vi "Read_Write_Local_table_Quick.vi"(3 "Mode":T1, 4 "String Values In":string[](array[string]), 5 "Ch names In":string[](array[string])) -> (0 "Numeric Values Out":dbl[](array[numeric]), 1 "String Values Out":string[](array[string]), 2 "Ch Names Out":string[](array[string]))   [LabVIEW 2020]
uses:
  ADAM Controls/Channel_names.ctl
  ADAM Controls/Quick_local_ADAM_Table.ctl
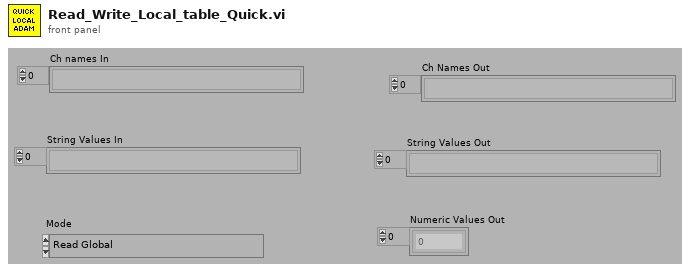
[diagram p1: front panel]
types:
  T1 = typedef "Quick_local_ADAM_Table.ctl" = enum16{"Read Global", "Load Global From ADAM Table", "Write Global"}
  T2 = typedef "Channel_names.ctl" = enum16{"Active Only", "Active + Off", "All Channels"}
  T3 = typedef "Ch_description_ADAM.ctl" = cluster{"Ch Name":string, "Type":T4, "Function":T5, "Ch State":T6, "Calibration type":T7, "A":dbl, "B":dbl, "C":dbl, "D":dbl, "Comments":string, "Address":T8, "String":string, "Duty":u16}
  T4 = typedef "Module_type_ADAM.ctl" = string
  T5 = typedef "Function_ADAM.ctl" = enum16{"Analogue Input", "Digital Input", "Event counter", "Event rate", "Analogue Output", "Digital Output", "Relay Output"}
  T6 = typedef "Channel_State.ctl" = enum16{"On", "Off", "Always On", "Always Off"}
  T7 = typedef "Calib_type_ADAM.ctl" = string
  T8 = typedef "Address.ctl" = cluster{"Main":i32, "Ch.":i32, "Sub":i32, "Port Name":string}
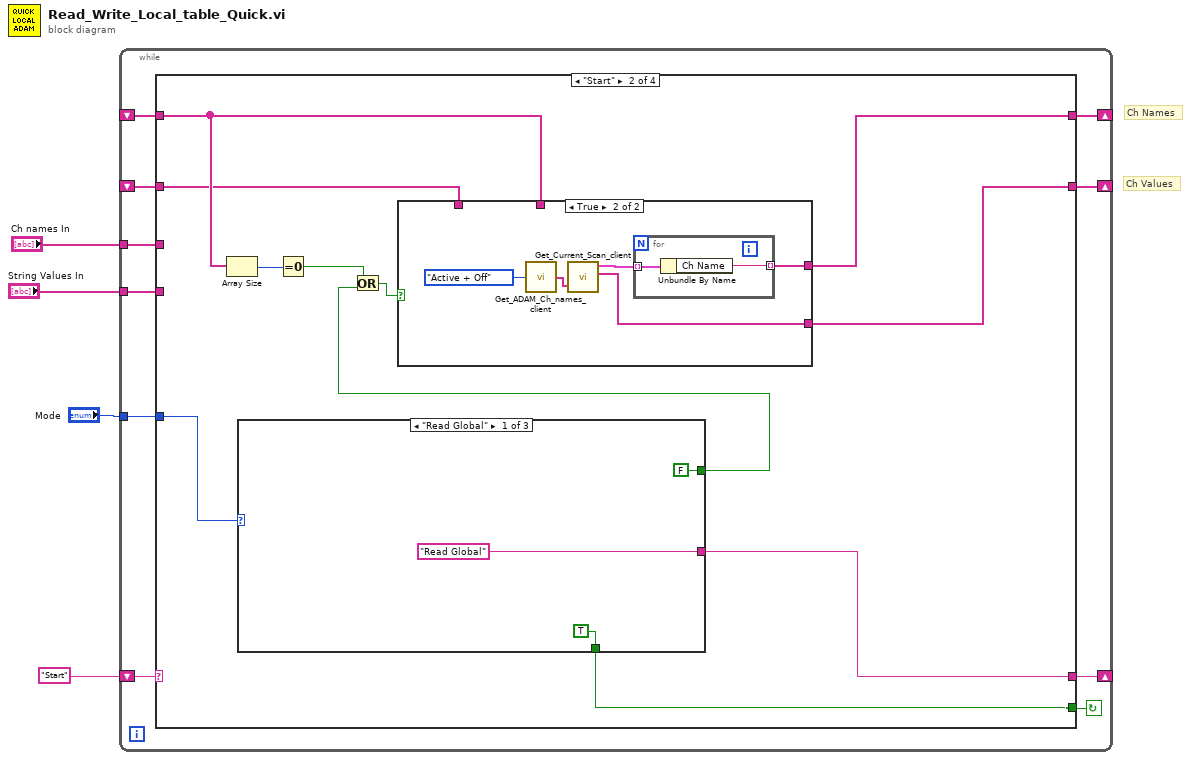
[diagram p0: block diagram]
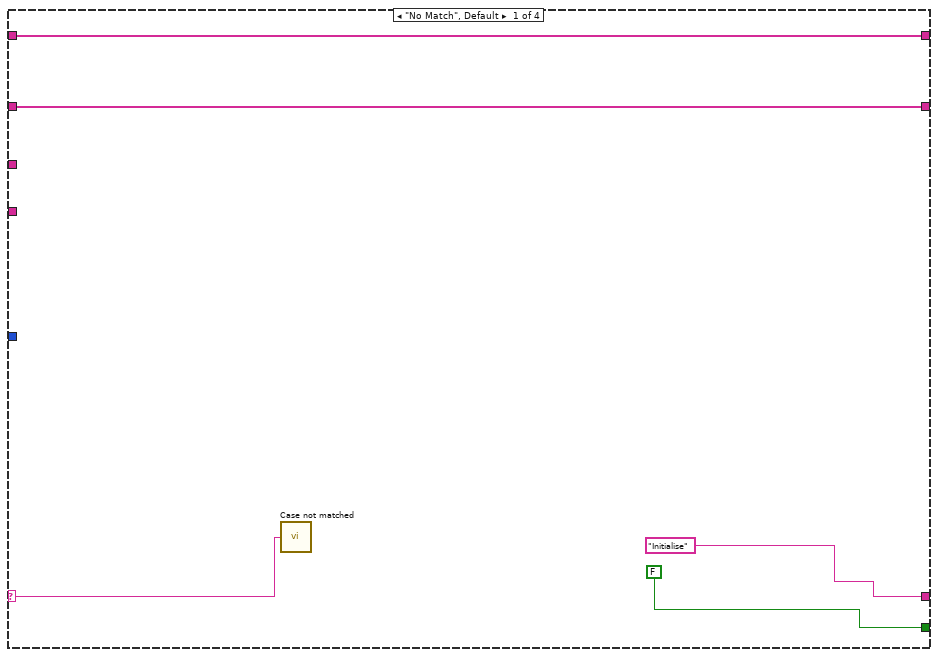
[diagram p2: hidden frame]
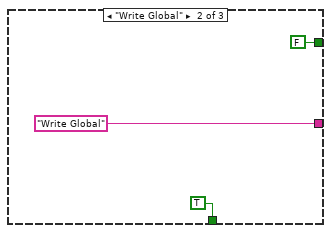
[diagram p4: hidden frame]
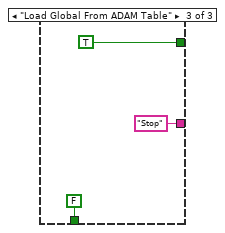
[diagram p5: hidden frame]
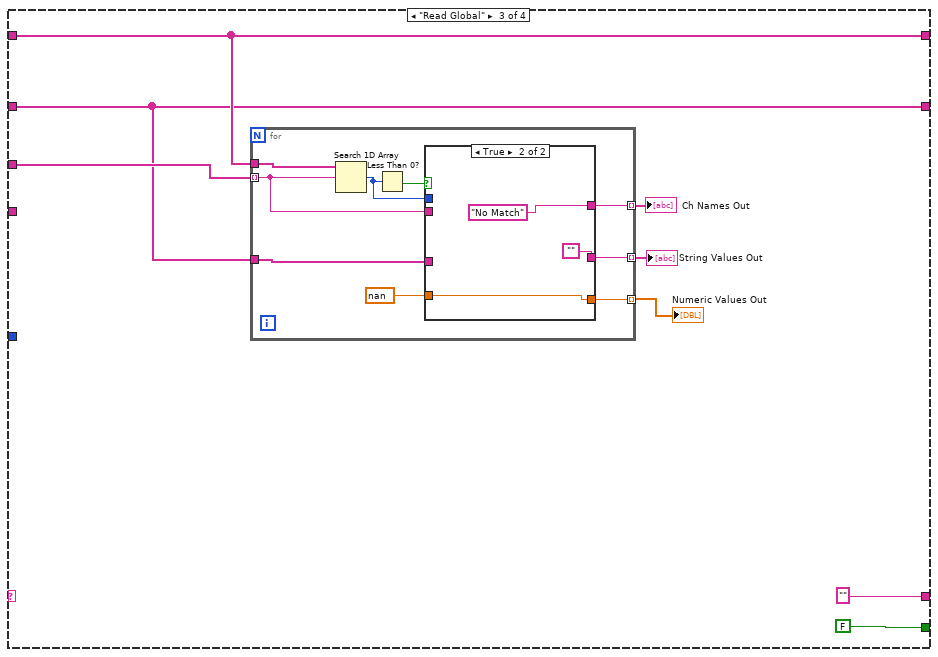
[diagram p6: hidden frame]
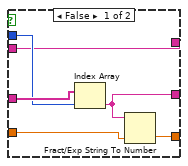
[diagram p7: hidden frame]
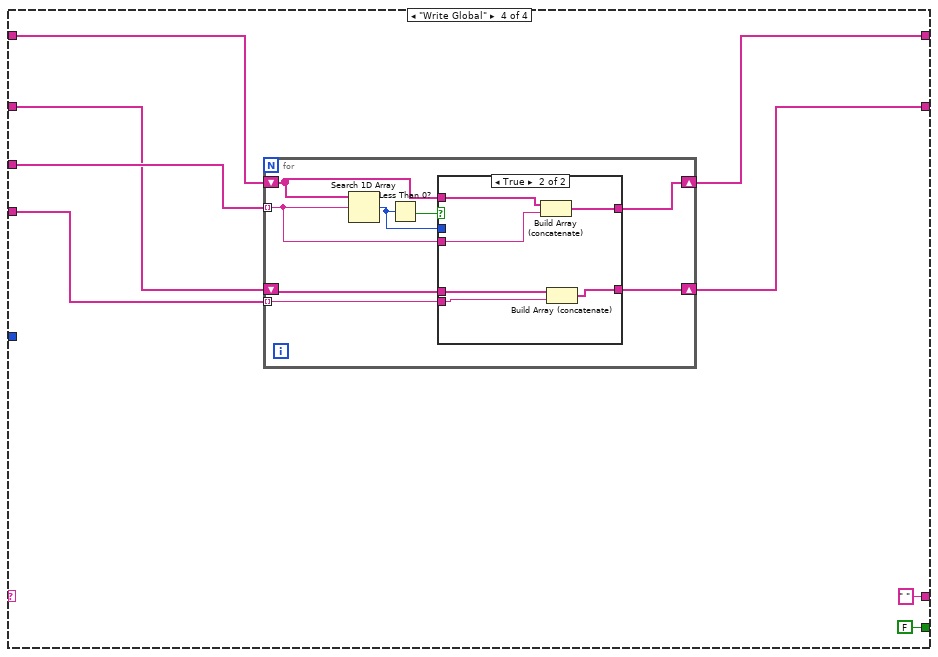
[diagram p8: hidden frame]
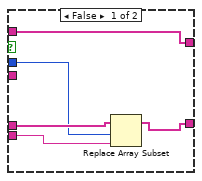
[diagram p9: hidden frame]
diagram:
  # "Ch Values"
  # "Ch Names"
  n1 = while {
    shift-left: "Start" -> [w12]
    shift-right: [w13] -> _
    shift-right: [w10] -> _
    shift-left: _ -> [w11]
    shift-right: [w9] -> _
    shift-left: _ -> [w7]
    tunnel: "Mode" -> [w8]
    tunnel: "Ch names In" -> [w6]
    tunnel: "String Values In" -> [w5]
    stop <- w14 continue-if-true
    n2 = case shown="\"Start\"" w12 {
      selector: w12 -> [w15 _ _ _]
      tunnel: [FALSE w20 FALSE FALSE] -> w14
      tunnel: ["Initialise" w21 "" " "] -> w13
      tunnel: w11 -> [w17 w23 w51 w82]
      tunnel: [w17 w30 w51 w80] -> w10
      tunnel: [w16 w29 w49 w77] -> w9
      tunnel: w8 -> [_ w28 _ _]
      tunnel: w7 -> [w16 w22 w49 w78]
      tunnel: w6 -> [_ _ w50 w81]
      tunnel: w5 -> [_ _ _ w79]
      frame "No Match", Default {
        n3 = call "Case not matched.vi"("Case Name not Matched"=w15) -> ()
      }
      frame "Start" {
        n4 = Array Size(array=w23) -> (size(s)=w27:i32)
        n5 = case shown="\"Read Global\"" w28 {
          tunnel: [FALSE FALSE TRUE] -> w26
          tunnel: ["Read Global" "Write Global" "Stop"] -> w21
          tunnel: [TRUE TRUE FALSE] -> w20
          frame "Read Global" {
          }
          frame "Write Global" {
          }
          frame "Load Global From ADAM Table" {
          }
        }
        n6 = Equal To 0?(x=w27) -> (x = 0?=w25:bool)
        n7 = Or(x=w25, y=w26) -> (x .or. y?=w24:bool)
        n8 = case shown="True" w24 {
          tunnel: [w32 w34] -> w30
          tunnel: [w31 w33] -> w29
          tunnel: w23 -> [w32 _]
          tunnel: w22 -> [w31 _]
          frame False {
          }
          frame True {
            n9 = call "Get_ADAM_Ch_names_client.vi"("Channel names set"=Channel_names."Active + Off") -> ("Ch names"=w36:string[])
            n10 = call "Get_Current_Scan_client.vi"("multipleChannels"=w36) -> ("Ch Description Array"=w37:T3[], "String values"=w33:string[])  [unwired: 2 in, 1 out]
            n11 = for {
              tunnel: w37 -> [w39] mode=indexing
              tunnel: [w38] -> w34 mode=indexing
              n12 = Unbundle By Name(w39) -> ("Ch Name"=w38:string)
            }
          }
        }
      }
      frame "Read Global" {
        n13 = for {
          tunnel: w50 -> [w64] mode=indexing
          tunnel: w49 -> [w62]
          tunnel: w51 -> [w61]
          tunnel: [w60] -> w52 mode=indexing
          tunnel: [w59] -> w53 mode=indexing
          tunnel: [w58] -> w54 mode=indexing
          n14 = Search 1D Array(1D array=w61, element=w64) -> (index of element=w63:i32)  [unwired: 1 in]
          n15 = Less Than 0?(x=w63) -> (x < 0?=w65:bool)
          n16 = case shown="True" w65 {
            tunnel: w64 -> [w69 _]
            tunnel: w62 -> [w71 _]
            tunnel: w63 -> [w70 _]
            tunnel: [w69 "No Match"] -> w60
            tunnel: [w68 ""] -> w59
            tunnel: [w67 w72] -> w58
            tunnel: nan ("default (0 DBL)") -> [w66 w72]
            frame False {
              n17 = Index Array(array=w71, index=w70) -> (element=w68:string)
              n18 = Fract/Exp String To Number(string=w68, default (0 dbl)=w66) -> (number=w67:dbl)  [unwired: 2 in, 1 out]
            }
            frame True {
            }
          }
        }
        "Ch Names Out" <- w52
        "String Values Out" <- w53
        "Numeric Values Out" <- w54
      }
      frame "Write Global" {
        n19 = for {
          tunnel: w81 -> [w88] mode=indexing
          shift-right: [w87] -> w80
          shift-left: w82 -> [w89]
          shift-right: [w84] -> w77
          shift-left: w78 -> [w86]
          tunnel: w79 -> [w85] mode=indexing
          n20 = Search 1D Array(1D array=w89, element=w88) -> (index of element=w83:i32)  [unwired: 1 in]
          n21 = Less Than 0?(x=w83) -> (x < 0?=w90:bool)
          n22 = case shown="True" w90 {
            tunnel: w89 -> [w91 w101]
            tunnel: w88 -> [_ w100]
            tunnel: [w91 w99] -> w87
            tunnel: w86 -> [w95 w98]
            tunnel: w85 -> [w93 w97]
            tunnel: [w92 w96] -> w84
            tunnel: w83 -> [w94 _]
            frame False {
              n23 = Replace Array Subset(array=w95, new element=w93, index=w94) -> (w92:string[])
            }
            frame True {
              n24 = Build Array (concatenate)(w101, w100) -> (w99:string[])
              n25 = Build Array (concatenate)(w98, w97) -> (w96:string[])
            }
          }
        }
      }
    }
  }
